vi "PH_SRDG645.contents.vi"   [LabVIEW 2014, in "PH_SRDG645.lvlib"]
uses:
  PH_SRDG645.lvlib
panel:
  # "This is the content vi for the SRDG645 Gate Delay Generator class"
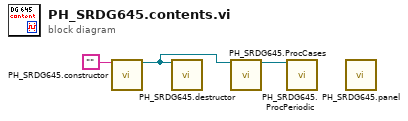
[diagram p0: block diagram]
diagram:
  n1 = call "PH_SRDG645.constructor.vi"("name"="") -> ("i ref out"=w1:refnum<vi>)  [unwired: 16 in, 2 out]
  n2 = call "PH_SRDG645.destructor.vi"("i ref in"=w1) -> ()  [unwired: 18 in, 1 out]
  n3 = call "PH_SRDG645.ProcCases.vi"("i ref in"=w1) -> ("i ref out"=w3:refnum<vi>)  [unwired: 16 in, 2 out]
  n4 = call "PH_SRDG645.ProcPeriodic.vi"("i ref in"=w3) -> ()  [unwired: 16 in, 3 out]
  n5 = call "PH_SRDG645.panel.vi"() -> ()  [unwired: 19 in, 1 out]
